vi "getTemplateFolderPath.vi"() -> (0 "Template Folder Path":path)   [LabVIEW 2017, in "shared.lvlib"]
uses:
  shared.lvlib
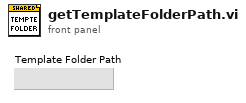
[diagram p1: front panel]
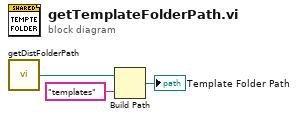
[diagram p0: block diagram]
diagram:
  n1 = call "getDistFolderPath.vi"() -> ("Dist Folder Path"=w3:path)
  n2 = Build Path(base path=w3, name or relative path="templates") -> (appended path=→"Template Folder Path":path)
